vi "Get DO On-Off Status.vi"(0 "reference in":refnum<class "DO.lvclass">, 5 "error in (no error)":errorcluster) -> (14 "reference out":refnum<class "DO.lvclass">, 18 "DO On/Off Status":bool, 19 "error out":errorcluster)   [LabVIEW 2017, in "DO.lvclass"]
uses:
  DO.lvclass
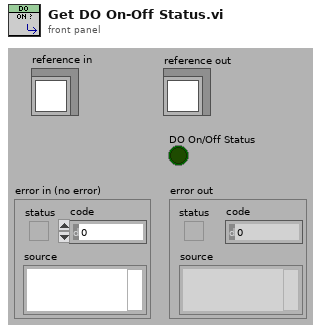
[diagram p1: front panel]
types:
  T1 = typedef "DO.lvclass/ObjectAttributes.ctl" = cluster{"DO Task":refnum<k21>, "DO Module Names (NI-Max Name)":string[], "Number of Channels Per DO Module":i32[], "DO Status":bool[], "Number of DO Modules":u32, "DO Status to Set":bool[], "DO On/Off Status":bool, "DO VI Reference":refnum<vi>, "Number of Total DO Channels":u32}
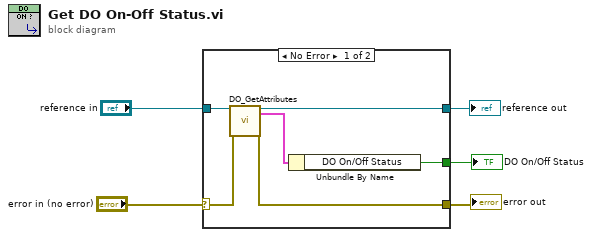
[diagram p0: block diagram]
diagram:
  n1 = case shown="No Error" "error in (no error)" {
    selector: "error in (no error)" -> [w11 w13]
    tunnel: [w9 w13] -> w4
    tunnel: [w7 w12] -> w2
    tunnel: "reference in" -> [w8 w12]
    tunnel: [w6 _] -> w1
    frame No Error {
      n2 = call "DO_GetAttributes.vi"("reference in"=w8, "error in (no error)"=w11) -> ("reference out"=w7:refnum<class "DO.lvclass">, "Data"=w10:T1, "error out"=w9:errorcluster)  [unwired: 14 in, 1 out]
      n3 = Unbundle By Name(w10) -> ("DO On/Off Status"=w6:bool)
    }
    frame Error {
    }
  }
  "error out" <- w4
  "reference out" <- w2
  "DO On/Off Status" <- w1
